vi "update.vi"(8 "error in (no error)":errorcluster, 10 "adapter executability":T1={"instrument"=TRUE, "trajectory"=TRUE, "scanHead"=TRUE, "DAQ"=TRUE, "imageAssembler"=TRUE, "dataCollection"=TRUE, "display"=TRUE, "analyser"=TRUE, "stimulator"=TRUE}, 11 "ImagingModeDL100901FlexTrajectory in":refnum<class "ImagingModeDL100901FlexTrajectory.lvclass">) -> (0 "error out":errorcluster, 3 "ImagingModeDL100901FlexTrajectory out":refnum<class "ImagingModeDL100901FlexTrajectory.lvclass">)   [LabVIEW 2010, in "ImagingModeDL100901FlexTrajectory.lvclass"]
uses:
  ImagingModeDL100901FlexTrajectory.lvclass
  ImagingModeDL090923Scaffold/ImagingModeDL090923Scaffold/adapter_executability_cluster.ctl
  ImagingModeDL091001Scaffold/ImagingModeDL091001Scaffold/ImagingModeDL091001Scaffold.lvclass
  ImagingModeDL100901FlexTrajectory.lvclass/ImagingModeDL100901FlexTrajectory.ctl
  Trajectory/GenericTrajectory/GenericTrajectory/GenericTrajectory.lvclass
  ScanHead/GenericScanHead/GenericScanHead/GenericScanHead.lvclass
  ImageAssembler/GenericImageAssembler/GenericImageAssembler/GenericImageAssembler.lvclass
  DataCollection/GenericDataCollection/GenericDataCollection/GenericDataCollection.lvclass
  ImagingModeDL090923Scaffold/ImagingModeDL090923Scaffold/ImagingModeDL090923Scaffold.lvclass
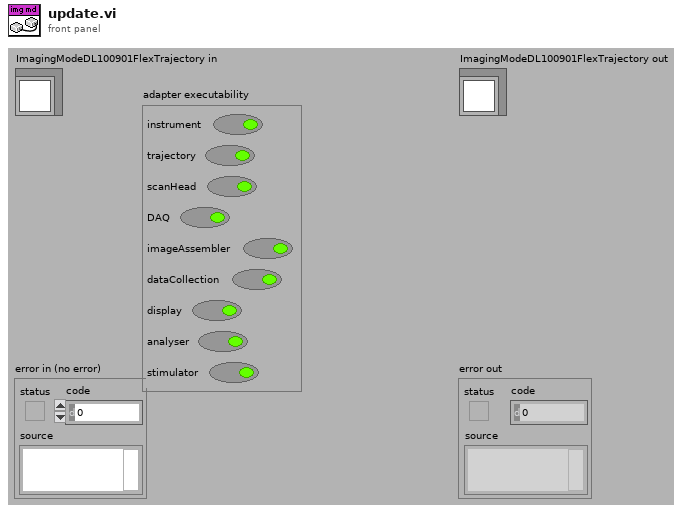
[diagram p1: front panel]
types:
  T1 = typedef "ImagingModeDL090923Scaffold.lvclass/adapter_executability_cluster.ctl" = cluster{"instrument":bool, "trajectory":bool, "scanHead":bool, "DAQ":bool, "imageAssembler":bool, "dataCollection":bool, "display":bool, "analyser":bool, "stimulator":bool}
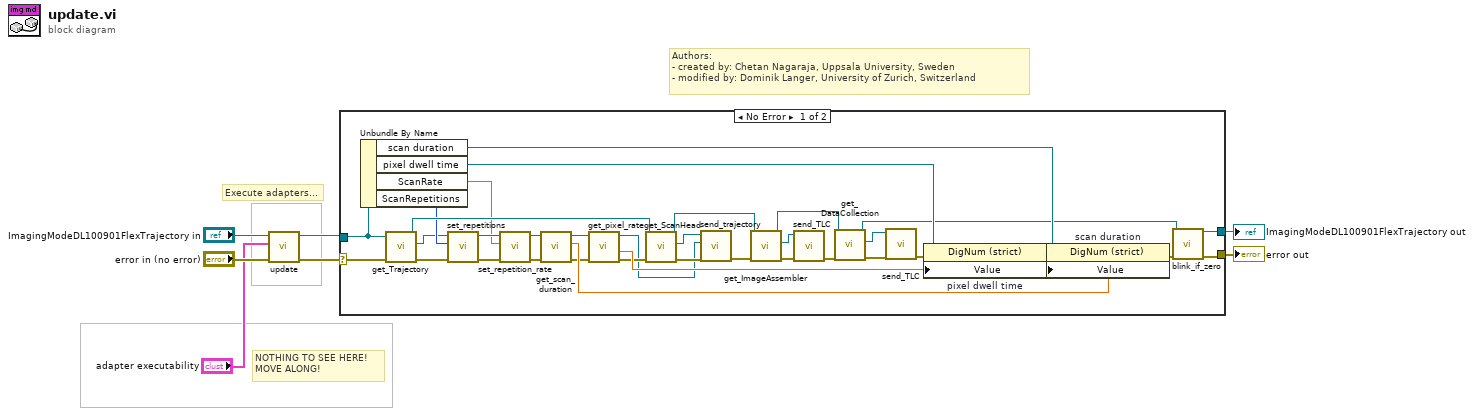
[diagram p0: block diagram]
diagram:
  # "NOTHING TO SEE HERE!\nMOVE ALONG!"
  # "Execute adapters..."
  # "Authors: \n- created by: Chetan Nagaraja, Uppsala University, Sweden\n- modified by: Dominik Langer, University of Zurich, Switzerland"
  n1 = call-parent "update.vi"("error in (no error)"="error in (no error)", "adapter executability"="adapter executability", "ScanModeDL090923Scaffold in"="ImagingModeDL100901FlexTrajectory in") -> ("error out"=w2:errorcluster, "ScanModeDL090923Scaffold out"=w5:refnum<class "ImagingModeDL100901FlexTrajectory.lvclass">)  [unwired: 7 in]
  n2 = case shown="No Error" w2 {
    selector: w2 -> [w39 w44]
    tunnel: [w11 w44] -> w3
    tunnel: [w10 w43] -> w4
    tunnel: w5 -> [w42 w43]
    frame No Error {
      n3 = Unbundle By Name(w42) -> ("scan duration"=w34:refnum<vi>, "pixel dwell time"=w35:refnum<vi>, "ScanRate"=w21:dbl[unit], "ScanRepetitions"=w24:i32)
      n4 = call-dynamic "get_Trajectory.vi"("error in (no error)"=w39, "ScanModeDL090923Scaffold in"=w42) -> ("error out"=w28:errorcluster, "Trajectory"=w13:refnum<class "GenericTrajectory.lvclass">, "ScanModeDL090923Scaffold out"=w27:refnum<class "ImagingModeDL100901FlexTrajectory.lvclass">)  [unwired: 7 out]
      n5 = call-dynamic "set_repetitions.vi"("error in (no error)"=w28, "repetitions"=w24, "GenericTrajectory in"=w13) -> ("error out"=w23:errorcluster, "GenericTrajectory out"=w22:refnum<class "GenericTrajectory.lvclass">)  [unwired: 7 in]
      n6 = call-dynamic "set_repetition_rate.vi"("error in (no error)"=w23, "repetition rate"=w21, "GenericTrajectory in"=w22) -> ("error out"=w18:errorcluster, "GenericTrajectory out"=w17:refnum<class "GenericTrajectory.lvclass">)  [unwired: 7 in]
      n7 = call-dynamic "get_scan_duration.vi"("error in (no error)"=w18, "GenericTrajectory in"=w17) -> ("error out"=w15:errorcluster, "scan duration"=w30:dbl[unit], "GenericTrajectory out"=w20:refnum<class "GenericTrajectory.lvclass">)  [unwired: 7 in]
      n8 = call-dynamic "get_pixel_rate.vi"("error in (no error)"=w15, "GenericTrajectory in"=w20) -> ("error out"=w16:errorcluster, "pixel dwell time"=w19:dbl[unit], "GenericTrajectory out"=w12:refnum<class "GenericTrajectory.lvclass">)  [unwired: 6 in, 1 out]
      n9 = call-dynamic "get_ScanHead.vi"("error in (no error)"=w16, "ScanModeDL090923Scaffold in"=w27) -> ("error out"=w26:errorcluster, "ScanHead"=w25:refnum<class "GenericScanHead.lvclass">, "ScanModeDL090923Scaffold out"=w32:refnum<class "ImagingModeDL100901FlexTrajectory.lvclass">)  [unwired: 4 in, 3 out]
      n10 = call-dynamic "send_trajectory.vi"("error in (no error)"=w26, "trajectory"=w12, "GenericScanHead in"=w25) -> ("error out"=w14:errorcluster)  [unwired: 8 out]
      n11 = call-dynamic "get_ImageAssembler.vi"("error in (no error)"=w14, "ScanModeDL090923Scaffold in"=w32) -> ("error out"=w38:errorcluster, "ImageAssembler"=w33:refnum<class "GenericImageAssembler.lvclass">, "ScanModeDL090923Scaffold out"=w41:refnum<class "ImagingModeDL100901FlexTrajectory.lvclass">)  [unwired: 4 in, 3 out]
      n12 = call-dynamic "send_TLC.vi"("error in (no error)"=w38, "GenericToplevelComponent in"=w33) -> ("error out"=w37:errorcluster)  [unwired: 8 in, 1 out]
      n13 = call-dynamic "get_DataCollection.vi"("error in (no error)"=w37, "ScanModeDL090923Scaffold in"=w41) -> ("error out"=w36:errorcluster, "DataCollection"=w40:refnum<class "GenericDataCollection.lvclass">, "ScanModeDL090923Scaffold out"=w8:refnum<class "ImagingModeDL100901FlexTrajectory.lvclass">)  [unwired: 4 in, 3 out]
      n14 = call-dynamic "send_TLC.vi"("error in (no error)"=w36, "GenericToplevelComponent in"=w40) -> ("error out"=w31:errorcluster)  [unwired: 8 in, 1 out]
      n15 = property on="pixel dwell time" class="DigNum (strict)"(reference=w35, error in=w31, "Value"=w19) -> (error out=w29:errorcluster)  [unwired: 1 out]
      n16 = property on="scan duration" class="DigNum (strict)"(reference=w34, error in=w29, "Value"=w30) -> (error out=w9:errorcluster)  [unwired: 1 out]
      n17 = call-dynamic "blink_if_zero.vi"("error in (no error)"=w9, "ImagingModeDL100901FlexTrajectory in"=w8) -> ("error out"=w11:errorcluster, "ImagingModeDL100901FlexTrajectory out"=w10:refnum<class "ImagingModeDL100901FlexTrajectory.lvclass">)  [unwired: 8 in]
    }
    frame Error {
    }
  }
  "error out" <- w3
  "ImagingModeDL100901FlexTrajectory out" <- w4
